vi "RP Transmit Data VISA.vi"(8 "Error In":errorcluster, 10 "Data":u32[](array[numeric]), 11 "VISA resource":refnum<visa-resource-name>) -> (0 "Error Out":errorcluster, 3 "VISA resource out":refnum<visa-resource-name>)   [LabVIEW 2015]
uses:
  RP Command.ctl
  RP Write Command VISA.vi
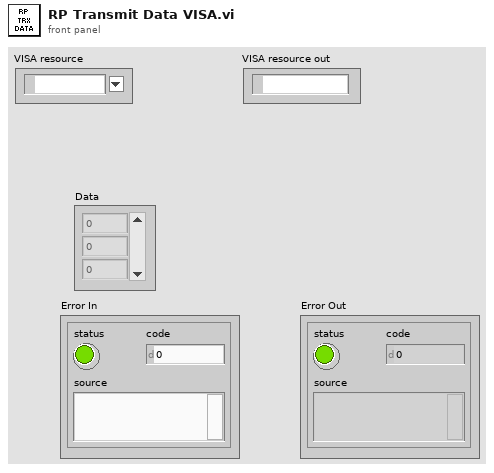
[diagram p1: front panel]
types:
  T1 = typedef "RP Command.ctl" = enum16{"Reset", "Read IDN", "Stop server", "Get status", "Get temperature", "Connect client", "Arm", "Software trigger", "Get whole buffer", "Get chunk", "System call", "Get config", "Set config", "Recieve data", "Play pattern", "Transmit data"}
  T2 = enum16{"big-endian, network order", "native, host order", "little-endian"}
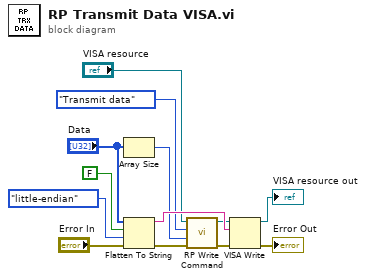
[diagram p0: block diagram]
diagram:
  n1 = Array Size(array="Data") -> (size(s)=w3:i32)
  n2 = Flatten To String(anything="Data", prepend array or string size? (T)=FALSE, byte order (0:big-endian, network order)=T2."little-endian", error in (no error)="Error In") -> (data string=w11:string, error out=w7:errorcluster)  [unwired: 1 out]
  n3 = call-poly "RP Write Command.vi"("Error In"=w7, "Command payload"=w3, "Command number"=RP_Command."Transmit data", "VISA resource"="VISA resource") -> ("Error Out"=w6:errorcluster, "VISA resource out"=w10:refnum<visa-resource-name>)  [unwired: 5 in, 1 out]
  n4 = VISA Write(VISA resource name=w10, write buffer=w11, error in (no error)=w6) -> (VISA resource name out=→"VISA resource out":refnum<visa-resource-name>, error out=→"Error Out":errorcluster)  [unwired: 1 out]
